vi "SIM Ros Coeffs.vi"() -> (0 "e32":dbl=7.414213562373095 format="%_20g", 1 "d":dbl=0.2928932188134525 format="%_20g")   [LabVIEW 2024]
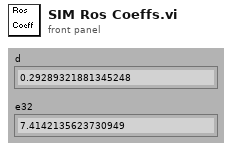
[diagram p1: front panel]
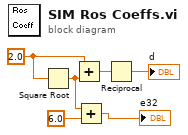
[diagram p0: block diagram]
diagram:
  w6 = 2.0 ("x")
  n1 = Square Root(x=w6) -> (sqrt(x)=w3:dbl)
  n2 = Add(x=w6, y=w3) -> (x+y=w5:dbl)
  n3 = Add(x=w3, y=6.0) -> (x+y=→"e32":dbl)
  n4 = Reciprocal(x=w5) -> (1/x=→"d":dbl)
